vi "FindVelScaleFactor.vi"(6 "V2 Velocity [V s-1]":dbl[](array[numeric])=[0.0, 0.0], 8 "V Velocity [V s-1]":dbl[](array[numeric])=[0.0, 0.0], 9 "Z Velocity [um s-1]":dbl[](array[numeric])=[0.0, 0.0], 10 "Y Velocity [um s-1]":dbl[](array[numeric])=[0.0, 0.0], 11 "X Velocity [um s-1]":dbl[](array[numeric])=[0.0, 0.0]) -> (0 "X_VelScaller":u32, 1 "V s-1_VelScaller":u32, 2 "Y_VelScaller":u32, 3 "Z_VelScaller":u32, 4 "V2 s-1_VelScaller":u32)   [LabVIEW 2023]
uses:
  User_Vi/Settings.vi
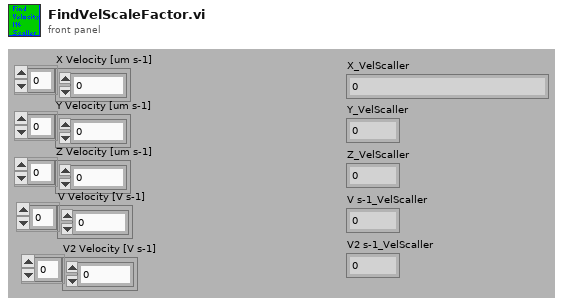
[diagram p1: front panel]
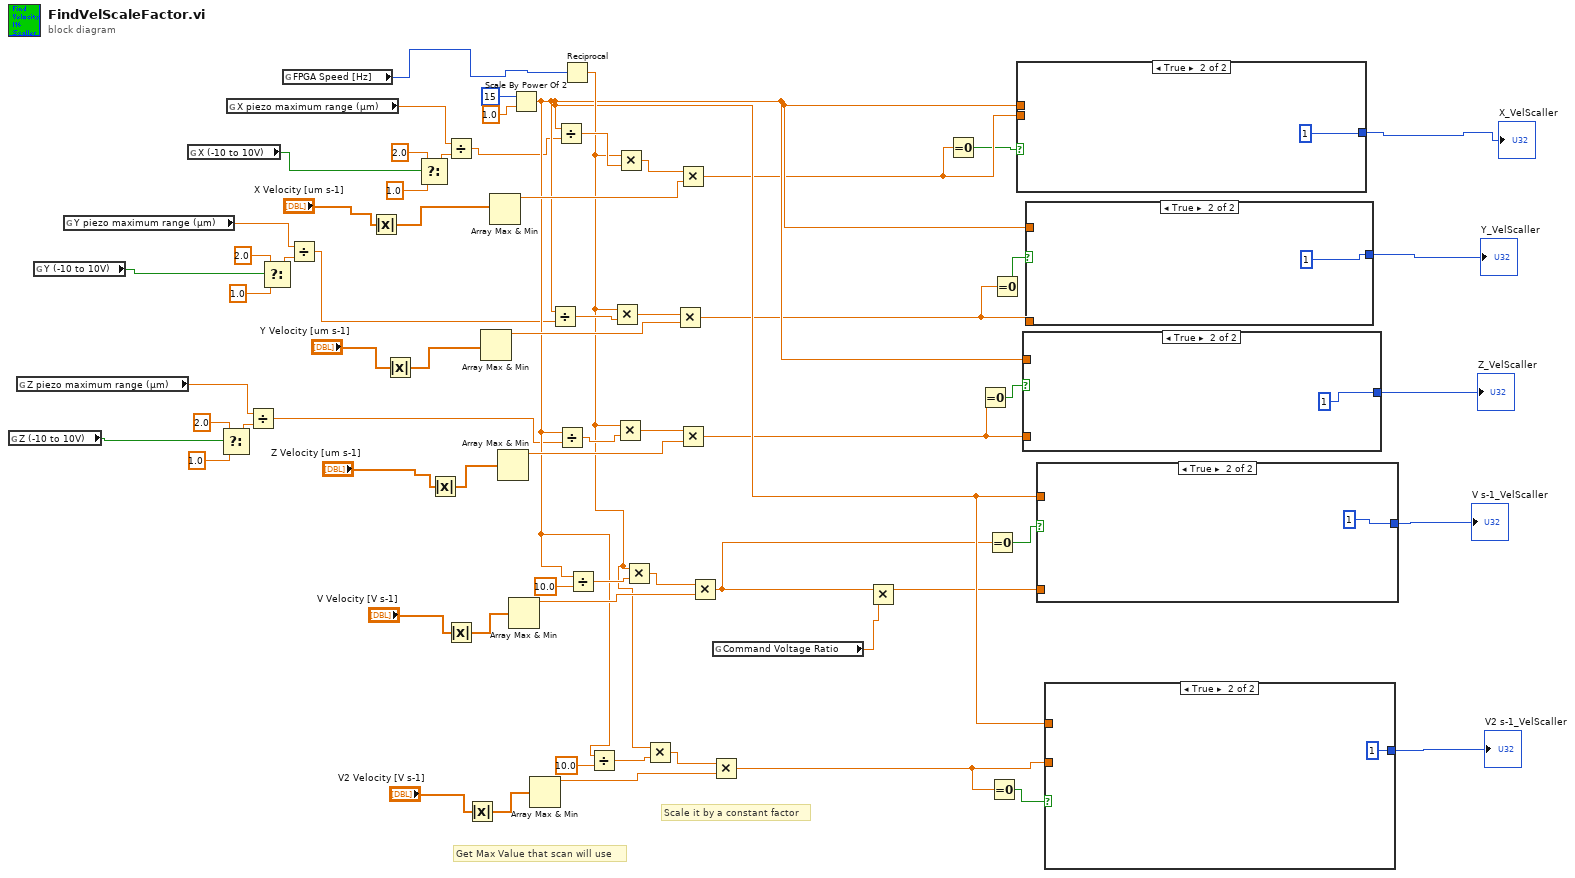
[diagram p0: block diagram]
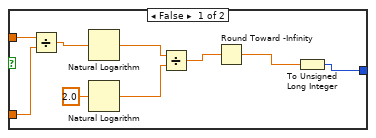
[diagram p2: hidden frame]
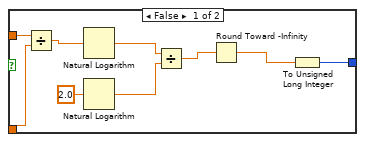
[diagram p3: hidden frame]
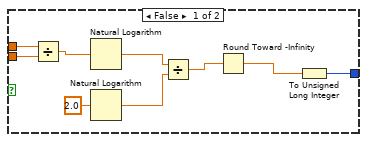
[diagram p4: hidden frame]
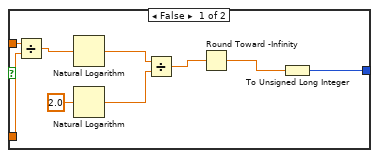
[diagram p5: hidden frame]
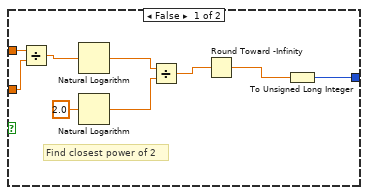
[diagram p6: hidden frame]
diagram:
  # "Scale it by a constant factor"
  # "Get Max Value that scan will use"
  n1 = global read "Settings.vi" "Z (-10 to 10V)"() -> (w2:bool)
  n2 = global read "Settings.vi" "Z piezo maximum range (µm)"() -> (w9:dbl)
  n3 = global read "Settings.vi" "Y (-10 to 10V)"() -> (w3:bool)
  n4 = global read "Settings.vi" "Y piezo maximum range (µm)"() -> (w7:dbl)
  n5 = global read "Settings.vi" "X (-10 to 10V)"() -> (w4:bool)
  n6 = Select(t=2.0, s=w2, f=1.0) -> (s? t:f=w12:dbl)
  n7 = global read "Settings.vi" "X piezo maximum range (µm)"() -> (w19:dbl)
  n8 = Divide(x=w9, y=w12) -> (x/y=w8:dbl)
  n9 = Select(t=2.0, s=w3, f=1.0) -> (s? t:f=w15:dbl)
  n10 = global read "Settings.vi" "FPGA Speed [Hz]"() -> (w5:i64)
  n11 = Divide(x=w7, y=w15) -> (x/y=w6:dbl)
  n12 = Absolute Value(x="X Velocity [um s-1]") -> (abs(x)=w51:dbl[])
  n13 = Absolute Value(x="Y Velocity [um s-1]") -> (abs(x)=w49:dbl[])
  n14 = Select(t=2.0, s=w4, f=1.0) -> (s? t:f=w20:dbl)
  n15 = Absolute Value(x="Z Velocity [um s-1]") -> (abs(x)=w47:dbl[])
  n16 = Divide(x=w19, y=w20) -> (x/y=w18:dbl)
  n17 = Absolute Value(x="V Velocity [V s-1]") -> (abs(x)=w45:dbl[])
  n18 = Absolute Value(x="V2 Velocity [V s-1]") -> (abs(x)=w40:dbl[])
  n19 = Array Max & Min(array=w49) -> (max value=w57:dbl)  [unwired: 3 out]
  n20 = Array Max & Min(array=w51) -> (max value=w60:dbl)  [unwired: 3 out]
  n21 = Array Max & Min(array=w47) -> (max value=w55:dbl)  [unwired: 3 out]
  n22 = Array Max & Min(array=w45) -> (max value=w53:dbl)  [unwired: 3 out]
  n23 = Scale By Power Of 2(n=i16 15, x=1.0) -> (x*2^n=w32:dbl)
  n24 = Array Max & Min(array=w40) -> (max value=w38:dbl)  [unwired: 3 out]
  n25 = Divide(x=w32, y=w6) -> (x/y=w63:dbl)
  n26 = Divide(x=w32, y=w18) -> (x/y=w64:dbl)
  n27 = Divide(x=w32, y=w8) -> (x/y=w62:dbl)
  n28 = Reciprocal(x=w5) -> (1/x=w34:dbl)
  n29 = Divide(x=w32, y=10.0) -> (x/y=w61:dbl)
  n30 = Divide(x=w32, y=10.0) -> (x/y=w36:dbl)
  n31 = Multiply(x=w34, y=w63) -> (x*y=w58:dbl)
  n32 = Multiply(x=w34, y=w62) -> (x*y=w56:dbl)
  n33 = Multiply(x=w34, y=w64) -> (x*y=w59:dbl)
  n34 = Multiply(x=w34, y=w61) -> (x*y=w54:dbl)
  n35 = Multiply(x=w34, y=w36) -> (x*y=w37:dbl)
  n36 = Multiply(x=w58, y=w57) -> (x*y=w26:dbl)
  n37 = Multiply(x=w59, y=w60) -> (x*y=w27:dbl)
  n38 = Multiply(x=w56, y=w55) -> (x*y=w25:dbl)
  n39 = Multiply(x=w54, y=w53) -> (x*y=w29:dbl)
  n40 = Multiply(x=w37, y=w38) -> (x*y=w31:dbl)
  n41 = global read "Settings.vi" "Command Voltage Ratio"() -> (w1:dbl)
  n42 = Multiply(x=w29, y=w1) -> (x*y=w21:dbl)
  n43 = Equal To 0?(x=w27) -> (x = 0?=w22:bool)
  n44 = Equal To 0?(x=w25) -> (x = 0?=w24:bool)
  n45 = Equal To 0?(x=w29) -> (x = 0?=w28:bool)
  n46 = Equal To 0?(x=w31) -> (x = 0?=w30:bool)
  n47 = Equal To 0?(x=w26) -> (x = 0?=w23:bool)
  n48 = case shown="True" w22 {
    tunnel: [w70 u32 1] -> w44
    tunnel: w32 -> [w69 _]
    tunnel: w27 -> [w68 _]
    frame False {
      n49 = Divide(x=w69, y=w68) -> (x/y=w76:dbl)
      n50 = Natural Logarithm(1:w76) -> (0:w73:dbl)
      n51 = Natural Logarithm(1:2.0 ("x")) -> (0:w74:dbl)
      n52 = Divide(x=w73, y=w74) -> (x/y=w72:dbl)
      n53 = Round Toward -Infinity(1:w72) -> (0:w71:dbl)
      n54 = To Unsigned Long Integer(number=w71) -> (unsigned 32bit integer=w70:u32)
    }
    frame True {
    }
  }
  "X_VelScaller" <- w44
  n55 = case shown="True" w24 {
    tunnel: [w80 u32 1] -> w42
    tunnel: w32 -> [w79 _]
    tunnel: w25 -> [w78 _]
    frame False {
      n56 = Divide(x=w79, y=w78) -> (x/y=w86:dbl)
      n57 = Natural Logarithm(1:w86) -> (0:w83:dbl)
      n58 = Natural Logarithm(1:2.0 ("x")) -> (0:w84:dbl)
      n59 = Divide(x=w83, y=w84) -> (x/y=w82:dbl)
      n60 = Round Toward -Infinity(1:w82) -> (0:w81:dbl)
      n61 = To Unsigned Long Integer(number=w81) -> (unsigned 32bit integer=w80:u32)
    }
    frame True {
    }
  }
  "Z_VelScaller" <- w42
  n62 = case shown="True" w23 {
    tunnel: [w90 u32 1] -> w43
    tunnel: w32 -> [w89 _]
    tunnel: w26 -> [w88 _]
    frame False {
      n63 = Divide(x=w89, y=w88) -> (x/y=w96:dbl)
      n64 = Natural Logarithm(1:w96) -> (0:w93:dbl)
      n65 = Natural Logarithm(1:2.0 ("x")) -> (0:w94:dbl)
      n66 = Divide(x=w93, y=w94) -> (x/y=w92:dbl)
      n67 = Round Toward -Infinity(1:w92) -> (0:w91:dbl)
      n68 = To Unsigned Long Integer(number=w91) -> (unsigned 32bit integer=w90:u32)
    }
    frame True {
    }
  }
  "Y_VelScaller" <- w43
  n69 = case shown="True" w28 {
    tunnel: [w100 u32 1] -> w41
    tunnel: w32 -> [w99 _]
    tunnel: w21 -> [w98 _]
    frame False {
      n70 = Divide(x=w99, y=w98) -> (x/y=w106:dbl)
      n71 = Natural Logarithm(1:w106) -> (0:w103:dbl)
      n72 = Natural Logarithm(1:2.0 ("x")) -> (0:w104:dbl)
      n73 = Divide(x=w103, y=w104) -> (x/y=w102:dbl)
      n74 = Round Toward -Infinity(1:w102) -> (0:w101:dbl)
      n75 = To Unsigned Long Integer(number=w101) -> (unsigned 32bit integer=w100:u32)
    }
    frame True {
    }
  }
  "V s-1_VelScaller" <- w41
  n76 = case shown="True" w30 {
    tunnel: [w116 u32 1] -> w33
    tunnel: w32 -> [w109 _]
    tunnel: w31 -> [w108 _]
    frame False {
      # "Find closest power of 2"
      n77 = Divide(x=w109, y=w108) -> (x/y=w110:dbl)
      n78 = Natural Logarithm(1:w110) -> (0:w113:dbl)
      n79 = Natural Logarithm(1:2.0 ("x")) -> (0:w112:dbl)
      n80 = Divide(x=w113, y=w112) -> (x/y=w114:dbl)
      n81 = Round Toward -Infinity(1:w114) -> (0:w115:dbl)
      n82 = To Unsigned Long Integer(number=w115) -> (unsigned 32bit integer=w116:u32)
    }
    frame True {
    }
  }
  "V2 s-1_VelScaller" <- w33
